vi "Martinas Aging Program v 1.1.vi"() -> ()   [LabVIEW 2011]
panel:
  out "Cell Settings Array":T1(array[cluster])=[{"Measure?"=TRUE, "Area (cm^2)"=0.0, "Cell Label"="", "Cell Description"="", "Time between scans (min)"=0.0, "Cell Position"=1, "Scan settings in queue"=0, "Sample holder"=1.0}, {"Measure?"=TRUE, "Area (cm^2)"=0.0, "Cell Label"="", "Cell Description"="", "Time between scans (min)"=0.0, "Cell Position"=2, "Scan settings in queue"=0, "Sample holder"=1.0}, {"Measure?"=TRUE, "Area (cm^2)"=0.0, "Cell Label"="", "Cell Description"="", "Time between scans (min)"=0.0, "Cell Position"=3, "Scan settings in queue"=0, "Sample holder"=1.0}, {"Measure?"=TRUE, "Area (cm^2)"=0.0, "Cell Label"="", "Cell Description"="", "Time between scans (min)"=0.0, "Cell Position"=4, "Scan settings in queue"=0, "Sample holder"=1.0}, {"Measure?"=TRUE, "Area (cm^2)"=0.0, "Cell Label"="", "Cell Description"="", "Time between scans (min)"=0.0, "Cell Position"=5, "Scan settings in queue"=0, "Sample holder"=1.0}, {"Measure?"=TRUE, "Area (cm^2)"=0.0, "Cell Label"="", "Cell Description"="", "Time between scans (min)"=0.0, "Cell Position"=6, "Scan settings in queue"=0, "Sample holder"=1.0}, {"Measure?"=TRUE, "Area (cm^2)"=0.0, "Cell Label"="", "Cell Description"="", "Time between scans (min)"=0.0, "Cell Position"=7, "Scan settings in queue"=0, "Sample holder"=1.0}, {"Measure?"=TRUE, "Area (cm^2)"=0.0, "Cell Label"="", "Cell Description"="", "Time between scans (min)"=0.0, "Cell Position"=8, "Scan settings in queue"=0, "Sample holder"=1.0}, {"Measure?"=TRUE, "Area (cm^2)"=0.0, "Cell Label"="", "Cell Description"="", "Time between scans (min)"=0.0, "Cell Position"=9, "Scan settings in queue"=0, "Sample holder"=1.0}, {"Measure?"=TRUE, "Area (cm^2)"=0.0, "Cell Label"="", "Cell Description"="", "Time between scans (min)"=0.0, "Cell Position"=10, "Scan settings in queue"=0, "Sample holder"=1.0}, {"Measure?"=TRUE, "Area (cm^2)"=0.0, "Cell Label"="", "Cell Description"="", "Time between scans (min)"=0.0, "Cell Position"=11, "Scan settings in queue"=0, "Sample holder"=1.0}, {"Measure?"=TRUE, "Area (cm^2)"=0.0, "Cell Label"="", "Cell Description"="", "Time between scans (min)"=0.0, "Cell Position"=12, "Scan settings in queue"=0, "Sample holder"=1.0}, {"Measure?"=TRUE, "Area (cm^2)"=0.0, "Cell Label"="", "Cell Description"="", "Time between scans (min)"=0.0, "Cell Position"=13, "Scan settings in queue"=0, "Sample holder"=1.0}, {"Measure?"=TRUE, "Area (cm^2)"=0.0, "Cell Label"="", "Cell Description"="", "Time between scans (min)"=0.0, "Cell Position"=14, "Scan settings in queue"=0, "Sample holder"=1.0}, {"Measure?"=TRUE, "Area (cm^2)"=0.0, "Cell Label"="", "Cell Description"="", "Time between scans (min)"=0.0, "Cell Position"=15, "Scan settings in queue"=0, "Sample holder"=1.0}, {"Measure?"=TRUE, "Area (cm^2)"=0.0, "Cell Label"="", "Cell Description"="", "Time between scans (min)"=0.0, "Cell Position"=16, "Scan settings in queue"=0, "Sample holder"=1.0}] {"Scan settings in queue" items=["Regular", "Inverted"]}
  in  "Tab Control":T2(tab)
  in  "Cell Settings Array 1":T3(array[cluster])=[{"Measure?"=TRUE, "Area (cm^2)"=0.0, "Cell Label"="", "Cell Description"="", "Time between scans (s)"=0.0, "Cell Position"=1, "Scan settings in queue"=0, "Sample holder"=1.0}, {"Measure?"=TRUE, "Area (cm^2)"=0.0, "Cell Label"="", "Cell Description"="", "Time between scans (s)"=0.0, "Cell Position"=2, "Scan settings in queue"=0, "Sample holder"=1.0}, {"Measure?"=TRUE, "Area (cm^2)"=0.0, "Cell Label"="", "Cell Description"="", "Time between scans (s)"=0.0, "Cell Position"=3, "Scan settings in queue"=0, "Sample holder"=1.0}, {"Measure?"=TRUE, "Area (cm^2)"=0.0, "Cell Label"="", "Cell Description"="", "Time between scans (s)"=0.0, "Cell Position"=4, "Scan settings in queue"=0, "Sample holder"=1.0}, {"Measure?"=TRUE, "Area (cm^2)"=0.0, "Cell Label"="", "Cell Description"="", "Time between scans (s)"=0.0, "Cell Position"=5, "Scan settings in queue"=0, "Sample holder"=1.0}, {"Measure?"=TRUE, "Area (cm^2)"=0.0, "Cell Label"="", "Cell Description"="", "Time between scans (s)"=0.0, "Cell Position"=6, "Scan settings in queue"=0, "Sample holder"=1.0}, {"Measure?"=TRUE, "Area (cm^2)"=0.0, "Cell Label"="", "Cell Description"="", "Time between scans (s)"=0.0, "Cell Position"=7, "Scan settings in queue"=0, "Sample holder"=1.0}, {"Measure?"=TRUE, "Area (cm^2)"=0.0, "Cell Label"="", "Cell Description"="", "Time between scans (s)"=0.0, "Cell Position"=8, "Scan settings in queue"=0, "Sample holder"=1.0}, {"Measure?"=TRUE, "Area (cm^2)"=0.0, "Cell Label"="", "Cell Description"="", "Time between scans (s)"=0.0, "Cell Position"=9, "Scan settings in queue"=0, "Sample holder"=1.0}, {"Measure?"=TRUE, "Area (cm^2)"=0.0, "Cell Label"="", "Cell Description"="", "Time between scans (s)"=0.0, "Cell Position"=10, "Scan settings in queue"=0, "Sample holder"=1.0}, {"Measure?"=TRUE, "Area (cm^2)"=0.0, "Cell Label"="", "Cell Description"="", "Time between scans (s)"=0.0, "Cell Position"=11, "Scan settings in queue"=0, "Sample holder"=1.0}, {"Measure?"=TRUE, "Area (cm^2)"=0.0, "Cell Label"="", "Cell Description"="", "Time between scans (s)"=0.0, "Cell Position"=12, "Scan settings in queue"=0, "Sample holder"=1.0}, {"Measure?"=TRUE, "Area (cm^2)"=0.0, "Cell Label"="", "Cell Description"="", "Time between scans (s)"=0.0, "Cell Position"=13, "Scan settings in queue"=0, "Sample holder"=1.0}, {"Measure?"=TRUE, "Area (cm^2)"=0.0, "Cell Label"="", "Cell Description"="", "Time between scans (s)"=0.0, "Cell Position"=14, "Scan settings in queue"=0, "Sample holder"=1.0}, {"Measure?"=TRUE, "Area (cm^2)"=0.0, "Cell Label"="", "Cell Description"="", "Time between scans (s)"=0.0, "Cell Position"=15, "Scan settings in queue"=0, "Sample holder"=1.0}, {"Measure?"=TRUE, "Area (cm^2)"=0.0, "Cell Label"="", "Cell Description"="", "Time between scans (s)"=0.0, "Cell Position"=16, "Scan settings in queue"=0, "Sample holder"=1.0}] {"Scan settings in queue" items=["Regular", "Inverted", "MartinaSettings"]}
  in  "Upload from Spreadsheet?":bool
  in  "Upload Spreadsheet path":path
  in  "Save to Spreadsheet?":bool
  in  "Save Spreadsheet Path":path
  in  "Cell Settings Array 2":T3(array[cluster])=[{"Measure?"=TRUE, "Area (cm^2)"=0.0, "Cell Label"="", "Cell Description"="", "Time between scans (s)"=0.0, "Cell Position"=1, "Scan settings in queue"=0, "Sample holder"=2.0}, {"Measure?"=TRUE, "Area (cm^2)"=0.0, "Cell Label"="", "Cell Description"="", "Time between scans (s)"=0.0, "Cell Position"=2, "Scan settings in queue"=0, "Sample holder"=2.0}, {"Measure?"=TRUE, "Area (cm^2)"=0.0, "Cell Label"="", "Cell Description"="", "Time between scans (s)"=0.0, "Cell Position"=3, "Scan settings in queue"=0, "Sample holder"=2.0}, {"Measure?"=TRUE, "Area (cm^2)"=0.0, "Cell Label"="", "Cell Description"="", "Time between scans (s)"=0.0, "Cell Position"=4, "Scan settings in queue"=0, "Sample holder"=2.0}, {"Measure?"=TRUE, "Area (cm^2)"=0.0, "Cell Label"="", "Cell Description"="", "Time between scans (s)"=0.0, "Cell Position"=5, "Scan settings in queue"=0, "Sample holder"=2.0}, {"Measure?"=TRUE, "Area (cm^2)"=0.0, "Cell Label"="", "Cell Description"="", "Time between scans (s)"=0.0, "Cell Position"=6, "Scan settings in queue"=0, "Sample holder"=2.0}, {"Measure?"=TRUE, "Area (cm^2)"=0.0, "Cell Label"="", "Cell Description"="", "Time between scans (s)"=0.0, "Cell Position"=7, "Scan settings in queue"=0, "Sample holder"=2.0}, {"Measure?"=TRUE, "Area (cm^2)"=0.0, "Cell Label"="", "Cell Description"="", "Time between scans (s)"=0.0, "Cell Position"=8, "Scan settings in queue"=0, "Sample holder"=2.0}, {"Measure?"=TRUE, "Area (cm^2)"=0.0, "Cell Label"="", "Cell Description"="", "Time between scans (s)"=0.0, "Cell Position"=9, "Scan settings in queue"=0, "Sample holder"=2.0}, {"Measure?"=TRUE, "Area (cm^2)"=0.0, "Cell Label"="", "Cell Description"="", "Time between scans (s)"=0.0, "Cell Position"=10, "Scan settings in queue"=0, "Sample holder"=2.0}, {"Measure?"=TRUE, "Area (cm^2)"=0.0, "Cell Label"="", "Cell Description"="", "Time between scans (s)"=0.0, "Cell Position"=11, "Scan settings in queue"=0, "Sample holder"=2.0}, {"Measure?"=TRUE, "Area (cm^2)"=0.0, "Cell Label"="", "Cell Description"="", "Time between scans (s)"=0.0, "Cell Position"=12, "Scan settings in queue"=0, "Sample holder"=2.0}, {"Measure?"=TRUE, "Area (cm^2)"=0.0, "Cell Label"="", "Cell Description"="", "Time between scans (s)"=0.0, "Cell Position"=13, "Scan settings in queue"=0, "Sample holder"=2.0}, {"Measure?"=TRUE, "Area (cm^2)"=0.0, "Cell Label"="", "Cell Description"="", "Time between scans (s)"=0.0, "Cell Position"=14, "Scan settings in queue"=0, "Sample holder"=2.0}, {"Measure?"=TRUE, "Area (cm^2)"=0.0, "Cell Label"="", "Cell Description"="", "Time between scans (s)"=0.0, "Cell Position"=15, "Scan settings in queue"=0, "Sample holder"=2.0}, {"Measure?"=TRUE, "Area (cm^2)"=0.0, "Cell Label"="", "Cell Description"="", "Time between scans (s)"=0.0, "Cell Position"=16, "Scan settings in queue"=0, "Sample holder"=2.0}] {"Scan settings in queue" items=["Regular", "Inverted", "MartinaSettings"]}
  in  "Upload Spreadsheet path 2":path
  in  "Upload from Spreadsheet? 2":bool
  in  "Save Spreadsheet Path 2":path
  in  "Save to Spreadsheet?  2":bool
  in  "Upload Spreadsheet path 3":path
  in  "Upload from Spreadsheet? 3":bool
  in  "Save Spreadsheet Path 3":path
  in  "Save to Spreadsheet?  3":bool
  in  "Cell Settings Array 3":T3(array[cluster])=[{"Measure?"=TRUE, "Area (cm^2)"=0.0, "Cell Label"="", "Cell Description"="", "Time between scans (s)"=0.0, "Cell Position"=1, "Scan settings in queue"=0, "Sample holder"=3.0}, {"Measure?"=TRUE, "Area (cm^2)"=0.0, "Cell Label"="", "Cell Description"="", "Time between scans (s)"=0.0, "Cell Position"=2, "Scan settings in queue"=0, "Sample holder"=3.0}, {"Measure?"=TRUE, "Area (cm^2)"=0.0, "Cell Label"="", "Cell Description"="", "Time between scans (s)"=0.0, "Cell Position"=3, "Scan settings in queue"=0, "Sample holder"=3.0}, {"Measure?"=TRUE, "Area (cm^2)"=0.0, "Cell Label"="", "Cell Description"="", "Time between scans (s)"=0.0, "Cell Position"=4, "Scan settings in queue"=0, "Sample holder"=3.0}, {"Measure?"=TRUE, "Area (cm^2)"=0.0, "Cell Label"="", "Cell Description"="", "Time between scans (s)"=0.0, "Cell Position"=5, "Scan settings in queue"=0, "Sample holder"=3.0}, {"Measure?"=TRUE, "Area (cm^2)"=0.0, "Cell Label"="", "Cell Description"="", "Time between scans (s)"=0.0, "Cell Position"=6, "Scan settings in queue"=0, "Sample holder"=3.0}, {"Measure?"=TRUE, "Area (cm^2)"=0.0, "Cell Label"="", "Cell Description"="", "Time between scans (s)"=0.0, "Cell Position"=7, "Scan settings in queue"=0, "Sample holder"=3.0}, {"Measure?"=TRUE, "Area (cm^2)"=0.0, "Cell Label"="", "Cell Description"="", "Time between scans (s)"=0.0, "Cell Position"=8, "Scan settings in queue"=0, "Sample holder"=3.0}, {"Measure?"=TRUE, "Area (cm^2)"=0.0, "Cell Label"="", "Cell Description"="", "Time between scans (s)"=0.0, "Cell Position"=9, "Scan settings in queue"=0, "Sample holder"=3.0}, {"Measure?"=TRUE, "Area (cm^2)"=0.0, "Cell Label"="", "Cell Description"="", "Time between scans (s)"=0.0, "Cell Position"=10, "Scan settings in queue"=0, "Sample holder"=3.0}, {"Measure?"=TRUE, "Area (cm^2)"=0.0, "Cell Label"="", "Cell Description"="", "Time between scans (s)"=0.0, "Cell Position"=11, "Scan settings in queue"=0, "Sample holder"=3.0}, {"Measure?"=TRUE, "Area (cm^2)"=0.0, "Cell Label"="", "Cell Description"="", "Time between scans (s)"=0.0, "Cell Position"=12, "Scan settings in queue"=0, "Sample holder"=3.0}, {"Measure?"=TRUE, "Area (cm^2)"=0.0, "Cell Label"="", "Cell Description"="", "Time between scans (s)"=0.0, "Cell Position"=13, "Scan settings in queue"=0, "Sample holder"=3.0}, {"Measure?"=TRUE, "Area (cm^2)"=0.0, "Cell Label"="", "Cell Description"="", "Time between scans (s)"=0.0, "Cell Position"=14, "Scan settings in queue"=0, "Sample holder"=3.0}, {"Measure?"=TRUE, "Area (cm^2)"=0.0, "Cell Label"="", "Cell Description"="", "Time between scans (s)"=0.0, "Cell Position"=15, "Scan settings in queue"=0, "Sample holder"=3.0}, {"Measure?"=TRUE, "Area (cm^2)"=0.0, "Cell Label"="", "Cell Description"="", "Time between scans (s)"=0.0, "Cell Position"=16, "Scan settings in queue"=0, "Sample holder"=3.0}] {"Scan settings in queue" items=["Regular", "Inverted", "MartinaSettings"]}
  in  "Cell Settings Array 4":T3(array[cluster])=[{"Measure?"=TRUE, "Area (cm^2)"=0.0, "Cell Label"="", "Cell Description"="", "Time between scans (s)"=0.0, "Cell Position"=1, "Scan settings in queue"=0, "Sample holder"=4.0}, {"Measure?"=TRUE, "Area (cm^2)"=0.0, "Cell Label"="", "Cell Description"="", "Time between scans (s)"=0.0, "Cell Position"=2, "Scan settings in queue"=0, "Sample holder"=4.0}, {"Measure?"=TRUE, "Area (cm^2)"=0.0, "Cell Label"="", "Cell Description"="", "Time between scans (s)"=0.0, "Cell Position"=3, "Scan settings in queue"=0, "Sample holder"=4.0}, {"Measure?"=TRUE, "Area (cm^2)"=0.0, "Cell Label"="", "Cell Description"="", "Time between scans (s)"=0.0, "Cell Position"=4, "Scan settings in queue"=0, "Sample holder"=4.0}, {"Measure?"=TRUE, "Area (cm^2)"=0.0, "Cell Label"="", "Cell Description"="", "Time between scans (s)"=0.0, "Cell Position"=5, "Scan settings in queue"=0, "Sample holder"=4.0}, {"Measure?"=TRUE, "Area (cm^2)"=0.0, "Cell Label"="", "Cell Description"="", "Time between scans (s)"=0.0, "Cell Position"=6, "Scan settings in queue"=0, "Sample holder"=4.0}, {"Measure?"=TRUE, "Area (cm^2)"=0.0, "Cell Label"="", "Cell Description"="", "Time between scans (s)"=0.0, "Cell Position"=7, "Scan settings in queue"=0, "Sample holder"=4.0}, {"Measure?"=TRUE, "Area (cm^2)"=0.0, "Cell Label"="", "Cell Description"="", "Time between scans (s)"=0.0, "Cell Position"=8, "Scan settings in queue"=0, "Sample holder"=4.0}, {"Measure?"=TRUE, "Area (cm^2)"=0.0, "Cell Label"="", "Cell Description"="", "Time between scans (s)"=0.0, "Cell Position"=9, "Scan settings in queue"=0, "Sample holder"=4.0}, {"Measure?"=TRUE, "Area (cm^2)"=0.0, "Cell Label"="", "Cell Description"="", "Time between scans (s)"=0.0, "Cell Position"=10, "Scan settings in queue"=0, "Sample holder"=4.0}, {"Measure?"=TRUE, "Area (cm^2)"=0.0, "Cell Label"="", "Cell Description"="", "Time between scans (s)"=0.0, "Cell Position"=11, "Scan settings in queue"=0, "Sample holder"=4.0}, {"Measure?"=TRUE, "Area (cm^2)"=0.0, "Cell Label"="", "Cell Description"="", "Time between scans (s)"=0.0, "Cell Position"=12, "Scan settings in queue"=0, "Sample holder"=4.0}, {"Measure?"=TRUE, "Area (cm^2)"=0.0, "Cell Label"="", "Cell Description"="", "Time between scans (s)"=0.0, "Cell Position"=13, "Scan settings in queue"=0, "Sample holder"=4.0}, {"Measure?"=TRUE, "Area (cm^2)"=0.0, "Cell Label"="", "Cell Description"="", "Time between scans (s)"=0.0, "Cell Position"=14, "Scan settings in queue"=0, "Sample holder"=4.0}, {"Measure?"=TRUE, "Area (cm^2)"=0.0, "Cell Label"="", "Cell Description"="", "Time between scans (s)"=0.0, "Cell Position"=15, "Scan settings in queue"=0, "Sample holder"=4.0}, {"Measure?"=TRUE, "Area (cm^2)"=0.0, "Cell Label"="", "Cell Description"="", "Time between scans (s)"=0.0, "Cell Position"=16, "Scan settings in queue"=0, "Sample holder"=4.0}] {"Scan settings in queue" items=["Regular", "Inverted", "MartinaSettings"]}
  in  "Upload Spreadsheet path 4":path
  in  "Upload from Spreadsheet? 4":bool
  in  "Save Spreadsheet Path 4":path
  in  "Save to Spreadsheet?  4":bool
  in  "Stop Scan":bool
  in  "Start Scan":bool
  out "Table":string[][](table)
  in  "Upload to the Queue":bool
  in  "Stop Scan 2":bool
  in  "Tab Control 4":enum32{"Page 1"}(tab)
  out "JV Curve":cluster{"Y":dbl[], "Y":dbl[]}[](graph)
  in  "Tab Control 2":enum32{"Page 1"}(tab)
  in  "Scan Settings JV":T4={"Light Intensity (Suns)"=1.0, "Stabilization Time (s)"=5.0, "Maximum Voltage (V)"=0.0, "Minimum Voltage (V)"=-1.0, "Range Options"=0, "Scan Direction"=TRUE, "Step Size (V)"=0.01, "Source Delay (s)"=0.15} {"Range Options" items=["Auto Range", "Semi-Auto Range", "100 uA", "1 mA", "10 mA", "100 mA", "1A"]}
  in  "Scan Setting Name":string
  in  "Add to Menu ring":bool
  in  "Show Scan settings":u16(ring) items=["Regular", "Inverted", "MartinaSettings"]
  in  "Delete from Menu Ring":bool
  in  "Tab Control 3":enum32{"Page 1"}(tab)
  out "Scan Settings JV 2":T4={"Light Intensity (Suns)"=1.0, "Stabilization Time (s)"=5.0, "Maximum Voltage (V)"=0.0, "Minimum Voltage (V)"=-1.0, "Range Options"=0, "Scan Direction"=TRUE, "Step Size (V)"=0.01, "Source Delay (s)"=0.15} {"Range Options" items=["Auto Range", "Semi-Auto Range", "100 uA", "1 mA", "10 mA", "100 mA", "1A"]}
  in  "Queue":T5(array[cluster]) {"Scan settings in queue" items=["Regular", "Inverted", "MartinaSettings"]; "Time of the last scan (s)" format="%<%H:%M:%S>t"; "When did you stick it in?" format="%<%H:%M:%S>t"; "Time to next scan (s)" format="%<%H:%M:%S>t"; "Time in rig (s)" format="%<%H:%M:%S>t"}
  out "TIMER":dbl format="%<%H:%M:%S>t"
  out "Username":string caption="Logged in as:"
  # "Cell Ageing"
  # "Time between Scans (s)"
  # "Area\n(cm^2)"
  # "Cell\nPosition"
  # "Sample\nHolder"
  # "On = working\nOff = not working"
  # "Label"
  # "Comment"
  # "Scan Settings"
  # "Time between Scans (s)"
  # "Area\n(cm^2)"
  # "Cell\nPosition"
  # "Sample\nHolder"
  # "On = working\nOff = not working"
  # "Label"
  # "Comment"
  # "Scan Settings"
  # "Time between Scans (s)"
  # "Area\n(cm^2)"
  # "Cell\nPosition"
  # "Sample\nHolder"
  # "On = working\nOff = not working"
  # "Label"
  # "Comment"
  # "Scan Settings"
  # "Time between Scans (s)"
  # "Area\n(cm^2)"
  # "Cell\nPosition"
  # "Sample\nHolder"
  # "On = working\nOff = not working"
  # "Label"
  # "Comment"
  # "Scan Settings"
  # "Time\n(s)"
  # "Light\nintensity"
  # "Cell\nLabel"
  # "Pixel\nNo."
  # "Scan\nNo."
  # "File\nPath"
  # "Area"
  # "Jsc"
  # "Voc"
  # "PCE"
  # "FF"
  # "Comment"
  # "LH (F)      HL (T)"
  # "LH (F)      HL (T)"
  # "Area\n(cm^2)"
  # "Scan\nwait (s)"
  # "Cell \nposition"
  # "Time in rig\n(hrs)"
  # "Time to next scan (hrs)"
  # "Scan\nnumber"
  # "Time\nZero"
  # "Time of \nlast scan"
  # "Sample\nHolder"
  # "On = working\nOff = not working"
  # "Label"
  # "Comment"
  # "Scan Settings"
  # "BASIC OPERATION:\n\nFill out the cell details for each cell in each sample holder on the \"Sample Holder #\" tabs. For easy data analysis later, the following format for the \n\"Comments\" box is recommended: [Cell maker]_[Date as yyyy-mm-dd]_[Experiment variation identifier], e.g. Martina_2014-02-29_Awesome Experiment. \nBe sure to compete all the information for each cell. If any boxes are blank, that cell won't be measured.\n\nGo to the \"Start/Stop Scan\" tab. Click the \"Initialise/Refresh Queue\" button. Check the \"Queue\" tab to make sure the the cell details have been added.\n\nOn the \"Start/Stop Scan\" tab click the \"Start Scan\" button. The cells in the queue will start to be measured.\n\n\n\nTO ADD/DELETE CUSTOM SCAN SETTINGS:\n\nGo to the \"Scan Settings\" tab.\n\nOn the left-hand pane, insert a new name into the \"Scan Setting Name\" box. Fill out the details in the pane and then press \"Add Settings\". \n\nExisting settings can be viewed by selecting the appropriate option on the right hand pane selection box on the \"Scan Settings\" tab. To delete the \nsettings currently being viewed, press the \"Delete Settings\" button.\n\n\n\nTO ADD/REMOVE/SWAP CELLS AND CONTINUE MEASUREMENT:\n\nGo to the \"Start/Stop Scan\" tab. Click the \"Stop Scan\" button. Wait for all the pixels on the current quad to finish measuring, plus all the pixels on the next\nquad in the queue. \n\nAdd/change the required cells and repeat \"Basic Operation\".\n\n\n\nADDITIONAL INFORMATION\n\nDuring the measurement, only the \"Stop Scan\" button is functional. No changes can be made whilst measurements are running. Any attempts to \npress other buttons during measurements will result in a program crash.\n\nYou cannot update the comments box once a cell has been uploaded to the queue."
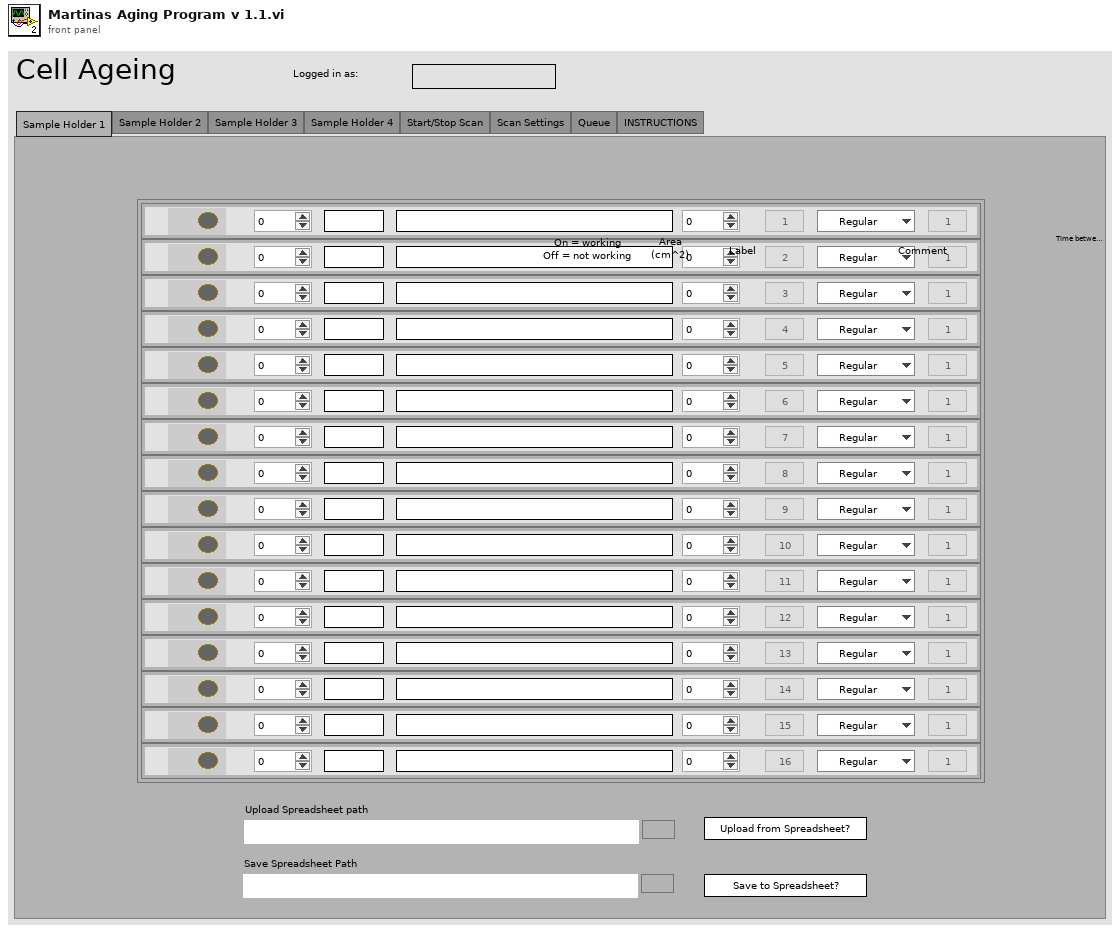
[diagram p1: front panel]
types:
  T1 = cluster{"Measure?":bool, "Area (cm^2)":dbl, "Cell Label":string, "Cell Description":string, "Time between scans (min)":dbl, "Cell Position":i32, "Scan settings in queue":u16, "Sample holder":dbl}[]
  T2 = enum32{"Sample Holder 1", "Sample Holder 2", "Sample Holder 3", "Sample Holder 4", "Start/Stop Scan", "Scan Settings", "Queue", "INSTRUCTIONS"}
  T3 = cluster{"Measure?":bool, "Area (cm^2)":dbl, "Cell Label":string, "Cell Description":string, "Time between scans (s)":dbl, "Cell Position":i32, "Scan settings in queue":u16, "Sample holder":dbl}[]
  T4 = cluster{"Light Intensity (Suns)":dbl, "Stabilization Time (s)":dbl, "Maximum Voltage (V)":dbl, "Minimum Voltage (V)":dbl, "Range Options":u16, "Scan Direction":bool, "Step Size (V)":dbl, "Source Delay (s)":dbl}
  T5 = cluster{"Measure?":bool, "Area (cm^2)":dbl, "Cell Label":string, "Cell Description":string, "Cell Position":i32, "Time in rig (s)":dbl, "Time to next scan (s)":dbl, "Scan number":dbl, "When did you stick it in?":dbl, "Time between scans (s)":dbl, "Time of the last scan (s)":dbl, "Scan settings in queue":u16, "Sample Holder":dbl}[]
  T6 = enum8{"Enabled", "Disabled", "Disabled and Grayed Out"}
  T7 = cluster{"Light Intensity (Suns)":dbl, "Stabilization Time (s)":dbl, "Maximum Voltage (V)":dbl, "Minimum Voltage (V)":dbl, "Range Options":u16, "Scan Direction\nDU (T), UD (F)":bool, "Step Size (V)":dbl, "Source Delay (s)":dbl}[]
  T8 = cluster{"Measure?":bool, "Area (cm^2)":dbl, "Cell Label":string, "Cell Description":string, "Cell Position":i32, "Time in rig (s)":dbl, "Time to next scan (s)":dbl, "Scan number":dbl, "When did you stick it in?":dbl, "Time between scans (s)":dbl, "Time of the last scan (s)":dbl, "Scan settings in queue":u16, "Sample Holder":dbl}
  T9 = cluster{"Light Intensity (Suns)":dbl, "Stabilization Time (s)":dbl, "Maximum Voltage (V)":dbl, "Minimum Voltage (V)":dbl, "Range Options":u16, "Scan Direction\nDU (T), UD (F)":bool, "Step Size (V)":dbl, "Source Delay (s)":dbl}
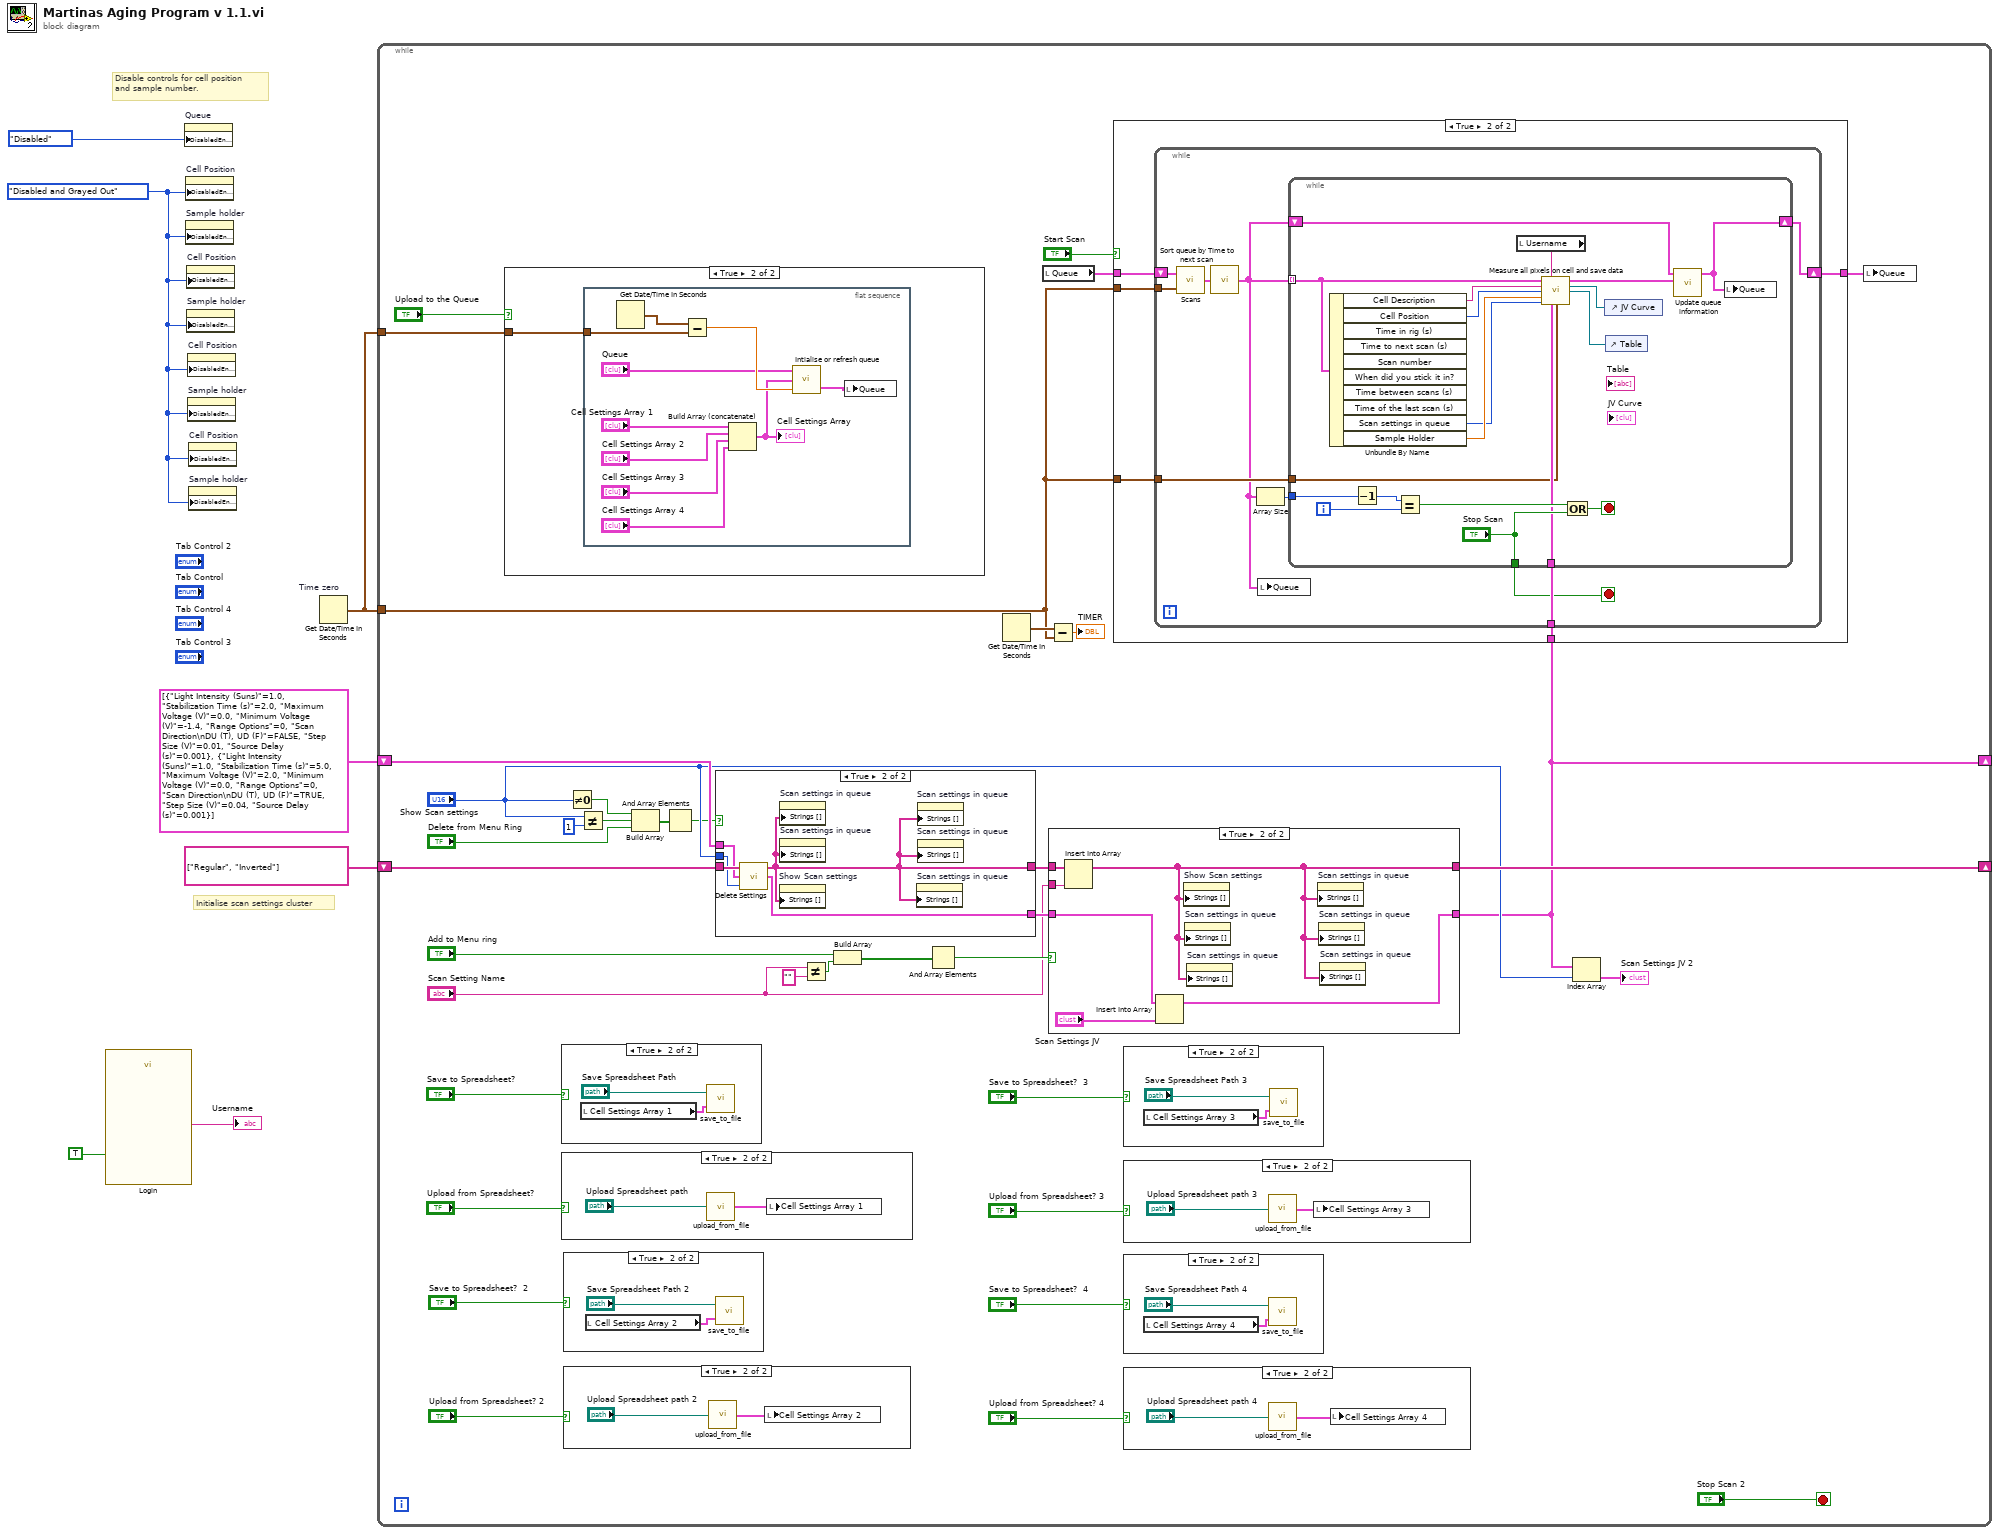
[diagram p0: block diagram]
diagram:
  w1 = T6."Disabled and Grayed Out" ("Disabled")
  # "Initialise scan settings cluster"
  # "Disable controls for cell position\nand sample number."
  n1 = call "Login"("Enable"=TRUE) -> ("Username"=→"Username":string)  [unwired: 16 in, 2 out]
  n2 = property on="Queue" class="Arr (strict)"("DisabledEnum"=T6."Disabled" ("Disabled")) -> ()  [unwired: 2 in, 2 out]
  n3 = property on="Cell Position" class="DigNum (strict)"("DisabledEnum"=w1) -> ()  [unwired: 2 in, 2 out]
  n4 = property on="Sample holder" class="DigNum (strict)"("DisabledEnum"=w1) -> ()  [unwired: 2 in, 2 out]
  n5 = property on="Cell Position" class="DigNum (strict)"("DisabledEnum"=w1) -> ()  [unwired: 2 in, 2 out]
  n6 = property on="Sample holder" class="DigNum (strict)"("DisabledEnum"=w1) -> ()  [unwired: 2 in, 2 out]
  n7 = property on="Cell Position" class="DigNum (strict)"("DisabledEnum"=w1) -> ()  [unwired: 2 in, 2 out]
  n8 = property on="Sample holder" class="DigNum (strict)"("DisabledEnum"=w1) -> ()  [unwired: 2 in, 2 out]
  n9 = property on="Cell Position" class="DigNum (strict)"("DisabledEnum"=w1) -> ()  [unwired: 2 in, 2 out]
  n10 = property on="Sample holder" class="DigNum (strict)"("DisabledEnum"=w1) -> ()  [unwired: 2 in, 2 out]
  n11 = Get Date/Time In Seconds "Time zero"() -> (seconds since 1Jan1904=w5:timestamp)
  n12 = while {
    tunnel: w5 -> [w41]
    shift-right: [w13] -> _
    shift-left: T7 [{"Light Intensity (Suns)"=1.0, "Stabilization Time (s)"=2.0, "Maximum Voltage (V)"=0.0, "Minimum Voltage (V)"=-1.4, "Range Options"=0, "Scan Direction\nDU (T), UD (F)"=FALSE, "Step Size (V)"=0.01, "Source Delay (s)"=0.001}, {"Light Intensity (Suns)"=1.0, "Stabilization Time (s)"=5.0, "Maximum Voltage (V)"=2.0, "Minimum Voltage (V)"=0.0, "Range Options"=0, "Scan Direction\nDU (T), UD (F)"=TRUE, "Step Size (V)"=0.04, "Source Delay (s)"=0.001}] ("JV curve scan settings 2") -> [w38]
    shift-right: [w40] -> _
    shift-left: string[] ["Regular", "Inverted"] ("Strings []") -> [w39]
    tunnel: w5 -> [w12]
    stop <- "Stop Scan 2" stop-if-true
    n13 = case shown="True" "Upload to the Queue" {
      tunnel: w41 -> [_ w106]
      frame False {
      }
      frame True {
        n14 = flat-sequence {
          tunnel: w106 -> [w116]
          frame #0 {
            n15 = Get Date/Time In Seconds() -> (seconds since 1Jan1904=w115:timestamp)
            n16 = Subtract(x=w115, y=w116) -> (x-y=w114:dbl)
            n17 = Build Array (concatenate)("Cell Settings Array 1", "Cell Settings Array 2", "Cell Settings Array 3", "Cell Settings Array 4") -> (w111:T3)
            "Cell Settings Array" <- w111
            n18 = call "Intialise or refresh queue.vi"("When did you stick it in?"=w114, "Cell Settings Array"=w111, "Queue in"="Queue") -> ("Queue out"=w110:T5)  [unwired: 1 in]
            n19 = local write "Queue"(w110) -> ()
          }
        }
      }
    }
    n20 = case shown="True" "Save to Spreadsheet?" {
      frame False {
      }
      frame True {
        n21 = local read "Cell Settings Array 1"() -> (w117:T3)
        n22 = call "save_to_file.vi"("Cell Settings Array 4"=w117, "Save Path"="Save Spreadsheet Path") -> ()  [unwired: 1 in]
      }
    }
    n23 = case shown="True" "Upload from Spreadsheet?" {
      frame False {
      }
      frame True {
        n24 = call "upload_from_file.vi"("Spreadsheet path"="Upload Spreadsheet path") -> ("Cell Settings Array 4"=w119:T1)
        n25 = local write "Cell Settings Array 1"(w119) -> ()
      }
    }
    n26 = case shown="True" "Save to Spreadsheet?  2" {
      frame False {
      }
      frame True {
        n27 = local read "Cell Settings Array 2"() -> (w53:T3)
        n28 = call "save_to_file.vi"("Cell Settings Array 4"=w53, "Save Path"="Save Spreadsheet Path 2") -> ()  [unwired: 1 in]
      }
    }
    n29 = case shown="True" "Upload from Spreadsheet? 2" {
      frame False {
      }
      frame True {
        n30 = call "upload_from_file.vi"("Spreadsheet path"="Upload Spreadsheet path 2") -> ("Cell Settings Array 4"=w55:T1)
        n31 = local write "Cell Settings Array 2"(w55) -> ()
      }
    }
    n32 = Not Equal To 0?(x="Show Scan settings") -> (x != 0?=w35:bool)
    n33 = Not Equal?(x="Show Scan settings", y=u16 1) -> (x != y?=w32:bool)
    n34 = Build Array(w35, w32, "Delete from Menu Ring") -> (w30:bool[])
    n35 = And Array Elements(Boolean array=w30) -> (logical AND=w29:bool)
    n36 = case shown="True" w29 {
      tunnel: w39 -> [w91 w97]
      tunnel: w38 -> [w92 w96]
      tunnel: "Show Scan settings" -> [_ w95]
      tunnel: [w91 w93] -> w37
      tunnel: [w92 w94] -> w36
      frame False {
      }
      frame True {
        n37 = call "Delete Settings.vi"("Scan settings"=w95, "JV curve scan settings"=w96, "Strings In"=w97) -> ("JV curve scan settings Out"=w94:T7, "Strings Out"=w93:string[])  [unwired: 1 out]
        n38 = property on="Show Scan settings" class="Ring (strict)"("Strings []"=w93) -> ()  [unwired: 2 in, 2 out]
        n39 = property on="Scan settings in queue" class="Ring (strict)"("Strings []"=w93) -> ()  [unwired: 2 in, 2 out]
        n40 = property on="Scan settings in queue" class="Ring (strict)"("Strings []"=w93) -> ()  [unwired: 2 in, 2 out]
        n41 = property on="Scan settings in queue" class="Ring (strict)"("Strings []"=w93) -> ()  [unwired: 2 in, 2 out]
        n42 = property on="Scan settings in queue" class="Ring (strict)"("Strings []"=w93) -> ()  [unwired: 2 in, 2 out]
        n43 = property on="Scan settings in queue" class="Ring (strict)"("Strings []"=w93) -> ()  [unwired: 2 in, 2 out]
      }
    }
    n44 = Not Equal?(x="Scan Setting Name", y="") -> (x != y?=w26:bool)
    n45 = Build Array("Add to Menu ring", w26) -> (w27:bool[])
    n46 = And Array Elements(Boolean array=w27) -> (logical AND=w24:bool)
    n47 = Get Date/Time In Seconds() -> (seconds since 1Jan1904=w21:timestamp)
    n48 = local read "Queue"() -> (w20:T5)
    n49 = Subtract(x=w21, y=w12) -> (x-y=→"TIMER":dbl)
    n50 = case shown="True" w24 {
      tunnel: w36 -> [w99 w105]
      tunnel: [w99 w104] -> w13
      tunnel: w37 -> [w98 w102]
      tunnel: [w98 w100] -> w40
      tunnel: "Scan Setting Name" -> [_ w101]
      frame False {
      }
      frame True {
        n51 = Insert Into Array(array=w102, new element=w101) -> (w100:string[])  [unwired: 1 in]
        n52 = Insert Into Array(array=w105, new element="Scan Settings JV") -> (w104:T7)  [unwired: 1 in]
        n53 = property on="Show Scan settings" class="Ring (strict)"("Strings []"=w100) -> ()  [unwired: 2 in, 2 out]
        n54 = property on="Scan settings in queue" class="Ring (strict)"("Strings []"=w100) -> ()  [unwired: 2 in, 2 out]
        n55 = property on="Scan settings in queue" class="Ring (strict)"("Strings []"=w100) -> ()  [unwired: 2 in, 2 out]
        n56 = property on="Scan settings in queue" class="Ring (strict)"("Strings []"=w100) -> ()  [unwired: 2 in, 2 out]
        n57 = property on="Scan settings in queue" class="Ring (strict)"("Strings []"=w100) -> ()  [unwired: 2 in, 2 out]
        n58 = property on="Scan settings in queue" class="Ring (strict)"("Strings []"=w100) -> ()  [unwired: 2 in, 2 out]
      }
    }
    n59 = case shown="True" "Start Scan" {
      tunnel: w20 -> [w57 w62]
      tunnel: w12 -> [_ w61]
      tunnel: [w57 w59] -> w11
      tunnel: w13 -> [_ w60]
      tunnel: w12 -> [_ w58]
      frame False {
      }
      frame True {
        n60 = while {
          tunnel: w61 -> [w70]
          tunnel: w60 -> [w68]
          shift-right: [w63] -> w59
          shift-left: w62 -> [w71]
          tunnel: w58 -> [w66]
          stop <- w65 stop-if-true
          n61 = call "Scans.vi"("Time zero (sec)"=w70, "Queue in"=w71) -> ("Queue out"=w69:T5)
          n62 = call "Sort queue by Time to next scan.vi"("Queue"=w69) -> ("Queue Out"=w64:T5)  [unwired: 4 in]
          n63 = Array Size(array=w64) -> (size(s)=w67:i32)
          n64 = local write "Queue"(w64) -> ()
          n65 = while {
            tunnel: w64 -> [w83] mode=indexing
            tunnel: w68 -> [w78]
            tunnel: w67 -> [w88]
            tunnel: w66 -> [w77]
            tunnel: ["Stop Scan"] -> w65
            shift-right: [w72] -> w63
            shift-left: w64 -> [w73]
            i -> [w90]
            stop <- w87 stop-if-true
            n66 = Unbundle By Name(w83) -> ("Cell Description"=w82:string, "Cell Position"=w81:i32, "Scan settings in queue"=w79:u16, "Sample Holder"=w80:dbl)  [unwired: 6 out]
            n67 = Decrement(x=w88) -> (x-1=w89:i32)
            n68 = Equal?(x=w89, y=w90) -> (x = y?=w86:bool)
            n69 = local read "Username"() -> (w84:string)
            n70 = Compound Arithmetic op=OR(w86, "Stop Scan") -> (w87:bool)
            n71 = control-ref of="JV Curve"() -> (w76:refnum<vi>)
            n72 = control-ref of="Table"() -> (w75:refnum<vi>)
            n73 = call "Measure all pixels on cell and save data.vi"("Cell details cluster in"=w83, "Username"=w84, "Cell Description"=w82, "XYGraph Refnum"=w76, "Cell position"=w81, "Tbl Refnum"=w75, "Sample Holder"=w80, "Scan settings in queue"=w79, "JV curve scan settings"=w78, "Time Zero"=w77) -> ("Cell details cluster out"=w74:T8)  [unwired: 4 in, 1 out]
            n74 = call "Update queue information.vi"("Cell details cluster"=w74, "Queue"=w73) -> ("Queue Out"=w72:T5)  [unwired: 3 in]
            n75 = local write "Queue"(w72) -> ()
          }
        }
      }
    }
    n76 = case shown="True" "Save to Spreadsheet?  3" {
      frame False {
      }
      frame True {
        n77 = local read "Cell Settings Array 3"() -> (w49:T3)
        n78 = call "save_to_file.vi"("Cell Settings Array 4"=w49, "Save Path"="Save Spreadsheet Path 3") -> ()  [unwired: 1 in]
      }
    }
    n79 = case shown="True" "Upload from Spreadsheet? 3" {
      frame False {
      }
      frame True {
        n80 = call "upload_from_file.vi"("Spreadsheet path"="Upload Spreadsheet path 3") -> ("Cell Settings Array 4"=w51:T1)
        n81 = local write "Cell Settings Array 3"(w51) -> ()
      }
    }
    n82 = case shown="True" "Save to Spreadsheet?  4" {
      frame False {
      }
      frame True {
        n83 = local read "Cell Settings Array 4"() -> (w45:T3)
        n84 = call "save_to_file.vi"("Cell Settings Array 4"=w45, "Save Path"="Save Spreadsheet Path 4") -> ()  [unwired: 1 in]
      }
    }
    n85 = case shown="True" "Upload from Spreadsheet? 4" {
      frame False {
      }
      frame True {
        n86 = call "upload_from_file.vi"("Spreadsheet path"="Upload Spreadsheet path 4") -> ("Cell Settings Array 4"=w47:T1)
        n87 = local write "Cell Settings Array 4"(w47) -> ()
      }
    }
    n88 = Index Array(array=w13, index="Show Scan settings") -> (element=→"Scan Settings JV 2":T9)
    n89 = local write "Queue"(w11) -> ()
  }
